vi "Check Parameters.vi"(8 "error in (no error)":errorcluster, 11 "Link in":refnum<class "Link.lvclass">) -> (0 "error out":errorcluster, 1 "dynamics valid":bool, 2 "kinematics valid":bool, 3 "Link out":refnum<class "Link.lvclass">)   [LabVIEW 2013, in "Link.lvclass"]
uses:
  Link.lvclass
  Link.lvclass/Link.ctl
  <vilib>/Analysis/_algsub.llb/Real Vector Norm.vi
  <vilib>/Analysis/NI_AALPro.lvlib
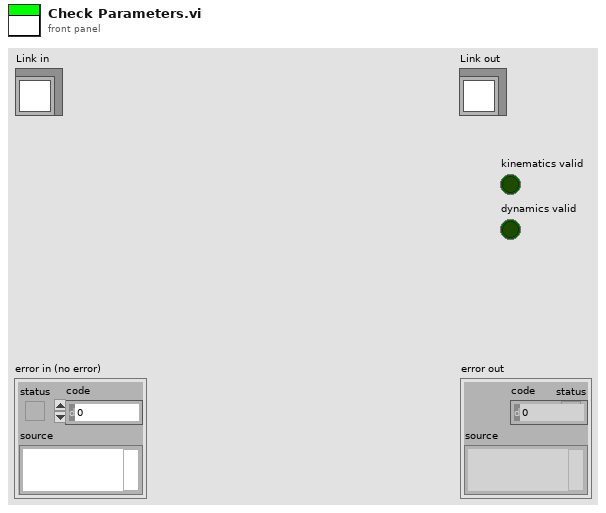
[diagram p1: front panel]
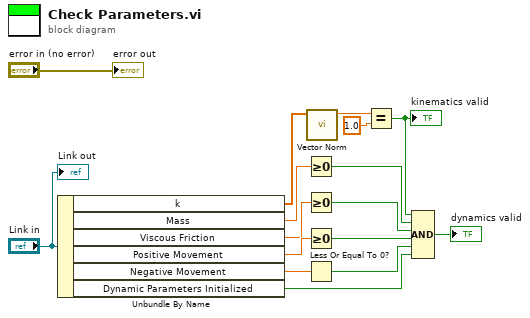
[diagram p0: block diagram]
diagram:
  n1 = Unbundle By Name("Link in") -> ("k"=w3:dbl[], "Mass"=w4:dbl, "Viscous Friction"=w5:dbl, "Positive Movement"=w6:dbl, "Negative Movement"=w7:dbl, "Dynamic Parameters Initialized"=w8:bool)
  n2 = Greater Or Equal To 0?(x=w4) -> (x >= 0?=w13:bool)
  n3 = Greater Or Equal To 0?(x=w5) -> (x >= 0?=w12:bool)
  n4 = Greater Or Equal To 0?(x=w6) -> (x >= 0?=w10:bool)
  n5 = Less Or Equal To 0?(x=w7) -> (x <= 0?=w11:bool)
  n6 = call-poly <vilib>:"Vector Norm.vi"("Input Vector"=w3) -> ("norm"=w1:dbl)  [unwired: 9 in, 1 out]
  n7 = Equal?(x=w1, y=1.0) -> (x = y?=w9:bool)
  "kinematics valid" <- w9
  n8 = Compound Arithmetic op=AND(w9, w13, w12, w10, w11, w8) -> (→"dynamics valid":bool)
  "error out" <- "error in (no error)"
  "Link out" <- "Link in"
